vi "Attach to Sub-pannel.vi"(8 "error in (no error)":errorcluster, 10 "Sub-pannel ref":refnum<vi>, 11 "Da Base in":refnum<class "Da Base.lvclass">) -> (0 "error out":errorcluster, 3 "Da Base out":refnum<class "Da Base.lvclass">)   [LabVIEW 2016, in "Da Base.lvclass"]
uses:
  Da Base.lvclass
  Da Base.lvclass/Da Base.ctl
  Read Front Panel ref.vi
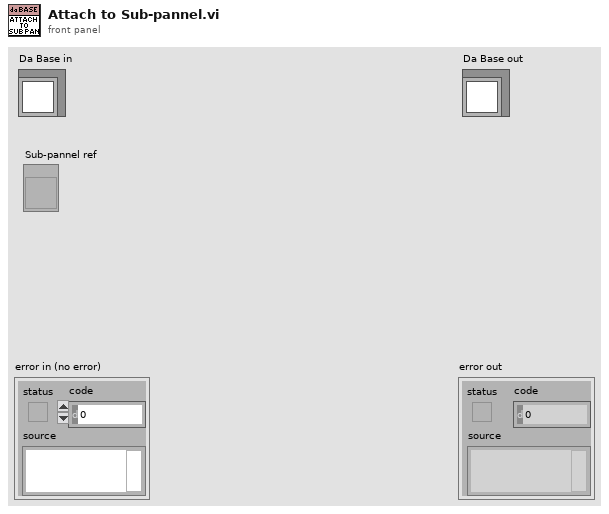
[diagram p1: front panel]
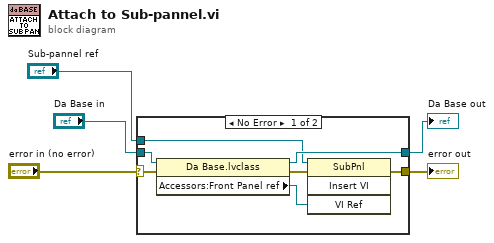
[diagram p0: block diagram]
diagram:
  n1 = case shown="No Error" "error in (no error)" {
    selector: "error in (no error)" -> [w12 w14]
    tunnel: [w6 w14] -> w4
    tunnel: [w10 w13] -> w2
    tunnel: "Da Base in" -> [w11 w13]
    tunnel: "Sub-pannel ref" -> [w8 _]
    frame No Error {
      n2 = property class="Da Base.lvclass"(reference=w11, error in=w12) -> (reference out=w10:refnum<class "Da Base.lvclass">, error out=w7:errorcluster, "Accessors:Front Panel ref"=w9:refnum<vi>)
      n3 = invoke class="SubPnl" method="Insert VI"(reference=w8, error in=w7, "VI Ref"=w9) -> (error out=w6:errorcluster)  [unwired: 1 in, 3 out]
    }
    frame Error {
    }
  }
  "error out" <- w4
  "Da Base out" <- w2
